vi "genTaskCommQueue.vi"(8 "error in (no error)":errorcluster, 11 "TaskName":string) -> (0 "error out":errorcluster, 3 "TaskCommQueue":refnum<queue>)   [LabVIEW 2010, in "pdbm_tasks.lvlib"]
uses:
  pdbm_tasks.lvlib
  UsrDefine/TaskRequest.ctl
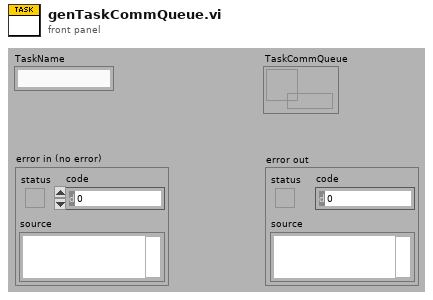
[diagram p1: front panel]
types:
  T1 = typedef "pdbm_tasks.lvlib/TaskRequest.ctl" = cluster{"Command":string, "Variant":variant}
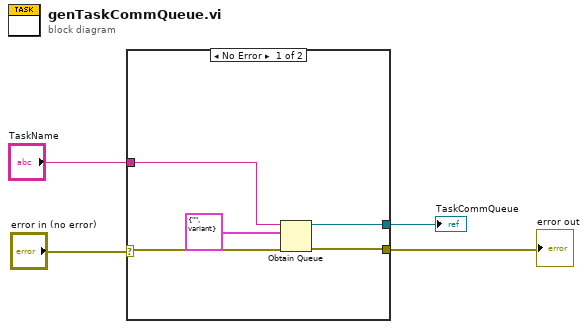
[diagram p0: block diagram]
diagram:
  n1 = case shown="No Error" "error in (no error)" {
    selector: "error in (no error)" -> [w6 w10]
    tunnel: [w9 w10] -> w2
    tunnel: [w8 _] -> w3
    tunnel: "TaskName" -> [w5 _]
    frame No Error {
      n2 = Obtain Queue(name (unnamed)=w5, element data type=T1 {"Command"="", "Variant"=variant} ("TaskRequest"), error in (no error)=w6) -> (queue out=w8:refnum<queue>, error out=w9:errorcluster)  [unwired: 2 in, 1 out]
    }
    frame Error {
    }
  }
  "TaskCommQueue" <- w3
  "error out" <- w2
